vi "Teardown Error.vi"(7 "Sender":refnum<class "Sender.lvclass">, 11 "Base Actor in":refnum<class "Base Actor.lvclass">) -> (3 "Base Actor out":refnum<class "Base Actor.lvclass">)   [LabVIEW 2020, in "jettl.lvlib" / "Actor.lvlib" / "Base Actor.lvclass"]
uses:
  Base Actor.lvclass
  Sender/Sender/Sender.lvclass
  Error/Error.lvlib
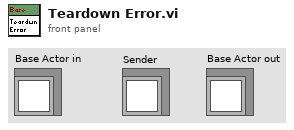
[diagram p1: front panel]
types:
  T1 = typedef "jettl.lvlib/Actor.lvlib/Error Info.ctl" = cluster{"Is Framework Error":bool, "Error":errorcluster}
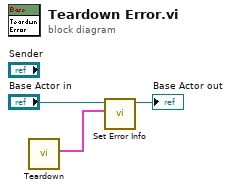
[diagram p0: block diagram]
diagram:
  n1 = call "Teardown.vi"() -> ("Error Info"=w1:T1)  [unwired: 11 in]
  n2 = call "Set Error Info.vi"("Error Info"=w1, "Base Actor in"="Base Actor in") -> ("Base Actor out"=→"Base Actor out":refnum<class "Base Actor.lvclass">)  [unwired: 9 in]
